vi "Append suffix.vi"(7 "Suffix":string, 8 "error in (no error)":errorcluster, 11 "Path":path) -> (0 "error out":errorcluster, 3 "Path out":path)   [LabVIEW 2021]
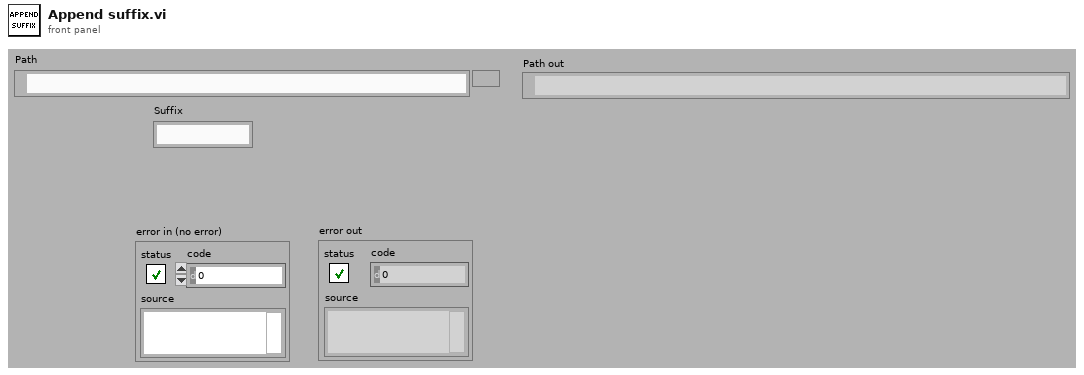
[diagram p1: front panel]
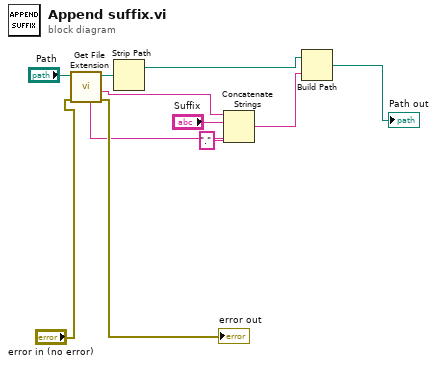
[diagram p0: block diagram]
diagram:
  n1 = call <vilib>:"Get File Extension.vi"("error in (no error)"="error in (no error)", "file"="Path") -> ("error out"=→"error out":errorcluster, "filename without extension"=w9:string, "dup file"=w8:path, "unmodified file extension"=w2:string)  [unwired: 5 in, 1 out]
  n2 = Strip Path(path=w8) -> (stripped path=w6:path)  [unwired: 1 out]
  n3 = Concatenate Strings(w9, "Suffix", "." ("string"), w2) -> (w7:string)
  n4 = Build Path(base path=w6, name or relative path=w7) -> (appended path=→"Path out":path)
